vi "Get Owning Pane of Control.vi"(8 "error in (no error)":errorcluster, 11 "GObj Refnum":refnum<vi>) -> (0 "error out":errorcluster, 1 "Pane Index":i32, 2 "Owning Pane":refnum<vi>, 3 "dup GObj Refnum":refnum<vi>)   [LabVIEW 2017, in "Front Panel Publisher.lvlib"]
uses:
  <vilib>/Utility/traverseref.llb/TRef TravTarget.ctl
  Front Panel Publisher.lvlib
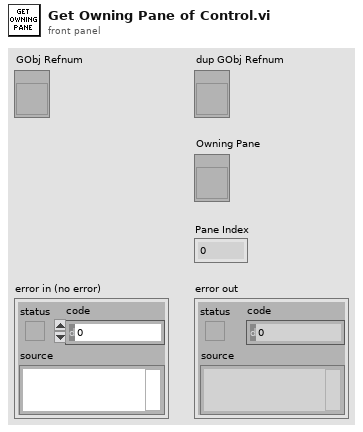
[diagram p1: front panel]
types:
  T1 = typedef "TRef TravTarget.ctl" = enum16{"FP", "BD", "Other"}
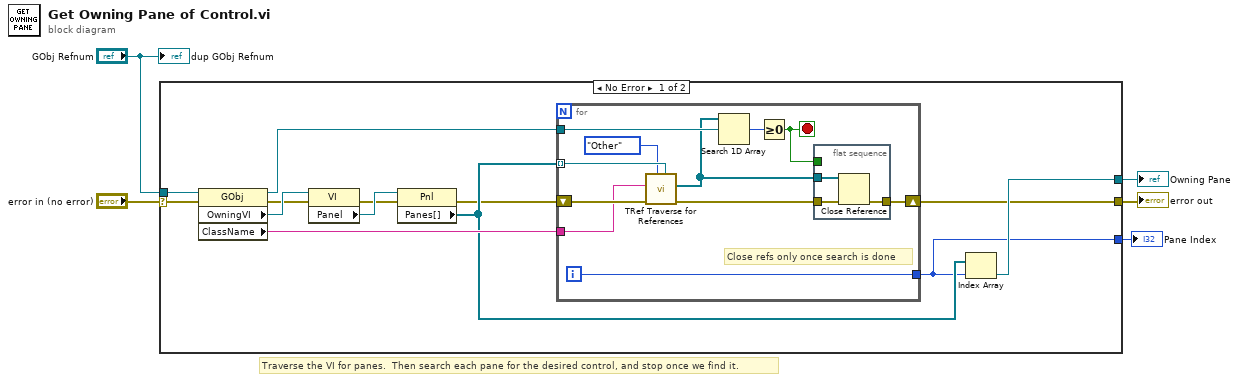
[diagram p0: block diagram]
diagram:
  # "Traverse the VI for panes.  Then search each pane for the desired control, and stop once we find it."
  n1 = case shown="No Error" "error in (no error)" {
    selector: "error in (no error)" -> [w18 w33]
    tunnel: [w7 w33] -> w4
    tunnel: "GObj Refnum" -> [w17 _]
    tunnel: [w8 _] -> w2
    tunnel: [w6 _] -> w1
    frame No Error {
      n2 = property class="GObj"(reference=w17, error in=w18) -> (reference out=w16:refnum<vi>, error out=w11:errorcluster, "OwningVI"=w14:refnum<vi>, "ClassName"=w15:string)
      n3 = property class="VI"(reference=w14, error in=w11) -> (error out=w10:errorcluster, "Panel"=w13:refnum<vi>)  [unwired: 1 out]
      n4 = property class="Pnl"(reference=w13, error in=w10) -> (error out=w9:errorcluster, "Panes[]"=w12:refnum<vi>[])  [unwired: 1 out]
      n5 = for {
        shift-right: [w23] -> w7
        shift-left: w9 -> [w29]
        tunnel: w12 -> [w28] mode=indexing
        tunnel: w16 -> [w26]
        tunnel: [w25] -> w6
        tunnel: w15 -> [w19]
        i -> [w25]
        stop <- w20 stop-if-true
        # "Close refs only once search is done"
        n6 = call <vilib>:"TRef Traverse for References.vi"("Other Refnum"=w28, "Traverse Target"=TRef_TravTarget."Other", "error in (no error)"=w29, "Class Name"=w19) -> ("error out"=w22:errorcluster, "References"=w21:refnum<vi>[])  [unwired: 4 in, 2 out]
        n7 = Search 1D Array(1D array=w21, element=w26) -> (index of element=w24:i32)  [unwired: 1 in]
        n8 = Greater Or Equal To 0?(x=w24) -> (x >= 0?=w20:bool)
        n9 = flat-sequence {
          tunnel: [w32] -> w23
          tunnel: w22 -> [w31]
          tunnel: w21 -> [w30]
          tunnel: w20 -> [_]
          frame #0 {
            n10 = Close Reference(reference=w30, error in (no error)=w31) -> (error out=w32:errorcluster)
          }
        }
      }
      n11 = Index Array(array=w12, index=w6) -> (element=w8:refnum<vi>)
    }
    frame Error {
    }
  }
  "error out" <- w4
  "Owning Pane" <- w2
  "Pane Index" <- w1
  "dup GObj Refnum" <- "GObj Refnum"
